vi "SLL DE Get Device Name from Physical Channel ID.vi"(8 "error in (no error)":errorcluster, 11 "GlobalChans":refnum<k21>[](array[refnum])) -> (0 "error out":errorcluster, 3 "Dev Names from Physical Channel":tag[](array[tag]))   [LabVIEW 2013]
doc: "Copyright © 2005, Soliton Technologies.\nAll rights reserved."
uses:
  <resource>/objmgr/daqmx.rc
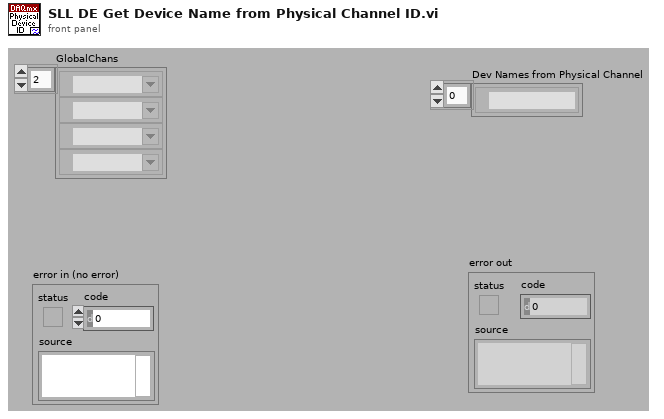
[diagram p1: front panel]
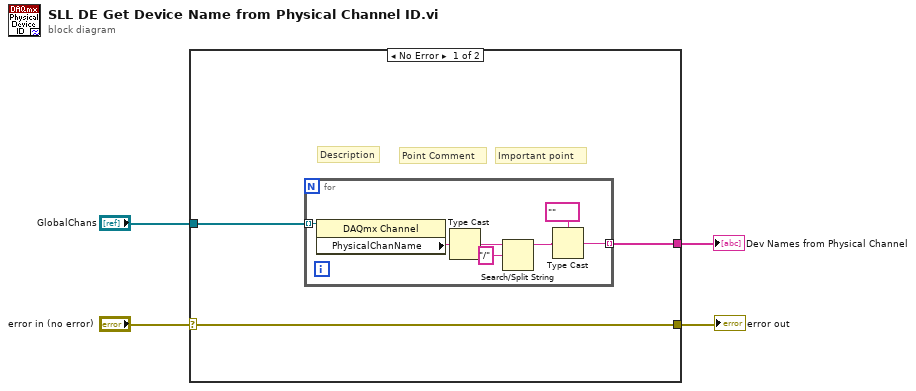
[diagram p0: block diagram]
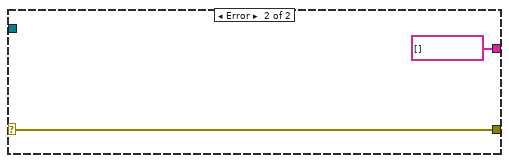
[diagram p2: hidden frame]
diagram:
  n1 = case shown="No Error" "error in (no error)" {
    selector: "error in (no error)" -> [w7 w16]
    tunnel: [w7 w16] -> w3
    tunnel: "GlobalChans" -> [w6 _]
    tunnel: [w5 tag[] []] -> w1
    frame No Error {
      # "Point Comment"
      # "Important point"
      # "Description"
      n2 = for {
        tunnel: w6 -> [w9] mode=indexing
        tunnel: [w8] -> w5 mode=indexing
        n3 = property class="DAQmx Channel"(reference=w9) -> ("PhysicalChanName"=w10:tag)  [unwired: 1 in, 2 out]
        n4 = Type Cast(x=w10) -> (*(type *) &x=w12:string)  [unwired: 1 in]
        n5 = Search/Split String(string=w12, search string/char (-)="/") -> (substring before match=w14:string)  [unwired: 1 in, 2 out]
        n6 = Type Cast(type=tag "", x=w14) -> (*(type *) &x=w8:tag)
      }
    }
    frame Error {
    }
  }
  "error out" <- w3
  "Dev Names from Physical Channel" <- w1
